vi "Get Team Ranking.vi"(11 "Needed Validations":u16) -> (3 "Ranked Teams":T1(array[cluster]))   [LabVIEW 2013]
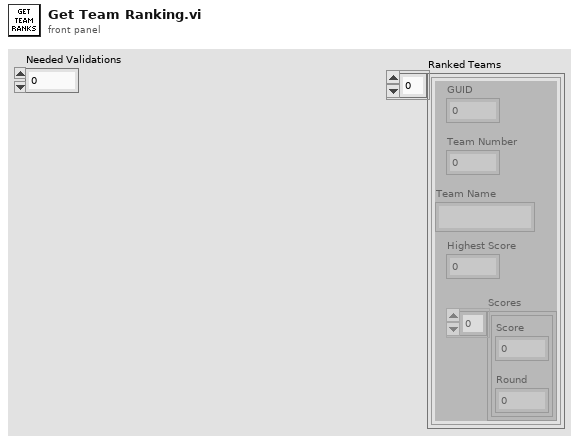
[diagram p1: front panel]
types:
  T1 = cluster{"GUID":u16, "Team Number":u16, "Team Name":string, "Highest Score":dbl, "Scores":cluster{"Score":dbl, "Round":u16}[]}[]
  T2 = cluster{"GUID":u16, "Team Number":u16, "Team Name":string, "Highest Score":dbl, "Scores":cluster{"Score":dbl, "Round":u16}[]}
  T3 = cluster{"Highest Score":dbl, "Scores":cluster{"Score":dbl, "Round":u16}[], "GUID":u16}[]
  T4 = typedef "ScoreList.ctl" = cluster{"ValidationCount":u16, "Score":T5}[]
  T5 = typedef "Full Score Entry.ctl" = cluster{"GUID":u16, "Score Mode Selector":u16, "Round Number":u16, "Full Score Entry":T6}
  T6 = typedef "ScoreEntry.ctl" = cluster{"Elements":cluster{"Name":string, "Value":string}[], "Score":dbl}
  T7 = cluster{"Highest Score":dbl, "Scores":cluster{"Score":dbl, "Round":u16}[], "GUID":u16}
  T8 = cluster{"Both":string, "Name":string, "GUID":u16, "Number":u16}
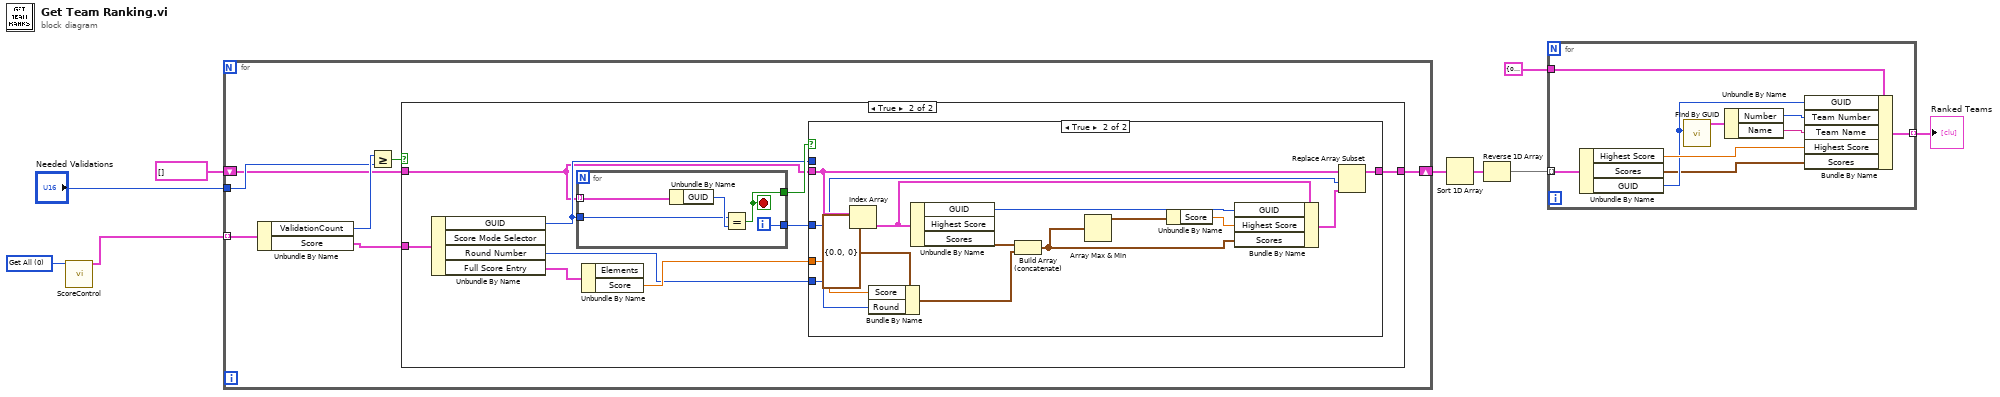
[diagram p0: block diagram]
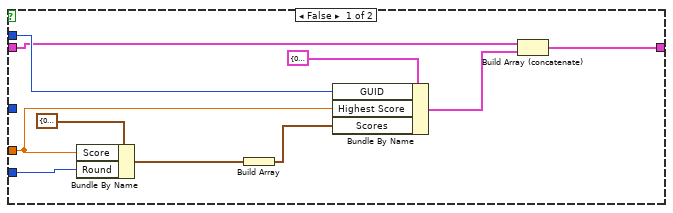
[diagram p3: hidden frame]
diagram:
  w2 = u16 0 items=["Get All", "Set", "Reset All", "Force Set"] ("Get/Set Mode Selector")
  n1 = call "ScoreControl.vi"("Get/Set Mode Selector"=w2) -> ("Scores"=w1:T4)  [unwired: 13 in, 1 out]
  n2 = for {
    tunnel: w1 -> [w16] mode=indexing
    tunnel: "Needed Validations" -> [w14]
    shift-right: [w10] -> w7
    shift-left: T3 [] -> [w11]
    n3 = Unbundle By Name(w16) -> ("ValidationCount"=w15:u16, "Score"=w12:T5)
    n4 = Greater Or Equal?(x=w15, y=w14) -> (x >= y?=w13:bool)
    n5 = case shown="True" w13 {
      tunnel: w12 -> [_ w26]
      tunnel: w11 -> [w17 w21]
      tunnel: [w17 w20] -> w10
      frame False {
      }
      frame True {
        n6 = Unbundle By Name(w26) -> ("GUID"=w24:u16, "Round Number"=w18:u16, "Full Score Entry"=w23:T6)  [unwired: 1 out]
        n7 = for {
          tunnel: w21 -> [w55] mode=indexing
          tunnel: w24 -> [w53]
          tunnel: [w52] -> w25
          tunnel: [w51] -> w19
          i -> [w51]
          stop <- w52 stop-if-true
          n8 = Unbundle By Name(w55) -> ("GUID"=w54:u16)
          n9 = Equal?(x=w53, y=w54) -> (x = y?=w52:bool)
        }
        n10 = Unbundle By Name(w23) -> ("Score"=w22:dbl)  [unwired: 1 out]
        n11 = case shown="True" w25 {
          tunnel: w24 -> [w35 _]
          tunnel: w22 -> [w29 w41]
          tunnel: w21 -> [w33 w47]
          tunnel: [w31 w44] -> w20
          tunnel: w19 -> [_ w46]
          tunnel: w18 -> [w28 w40]
          frame False {
            n12 = Bundle By Name(cluster=cluster{"Score":dbl, "Round":u16} {"Score"=0.0, "Round"=0}, "Score"=w29, "Round"=w28) -> (w27:cluster{"Score":dbl, "Round":u16})
            n13 = Build Array(w27) -> (w34:cluster{"Score":dbl, "Round":u16}[])
            n14 = Bundle By Name(cluster=T7 {"Highest Score"=0.0, "Scores"=[], "GUID"=0}, "GUID"=w35, "Highest Score"=w29, "Scores"=w34) -> (w32:T7)
            n15 = Build Array (concatenate)(w33, w32) -> (w31:T3)
          }
          frame True {
            n16 = Index Array(array=w47, index=w46) -> (element=w50:T7)
            n17 = Bundle By Name(cluster=cluster{"Score":dbl, "Round":u16} {"Score"=0.0, "Round"=0}, "Score"=w41, "Round"=w40) -> (w42:cluster{"Score":dbl, "Round":u16})
            n18 = Unbundle By Name(w50) -> ("GUID"=w49:u16, "Scores"=w37:cluster{"Score":dbl, "Round":u16}[])  [unwired: 1 out]
            n19 = Build Array (concatenate)(w37, w42) -> (w48:cluster{"Score":dbl, "Round":u16}[])
            n20 = Array Max & Min(array=w48) -> (max value=w39:cluster{"Score":dbl, "Round":u16})  [unwired: 3 out]
            n21 = Unbundle By Name(w39) -> ("Score"=w38:dbl)
            n22 = Bundle By Name(cluster=w50, "GUID"=w49, "Highest Score"=w38, "Scores"=w48) -> (w45:T7)
            n23 = Replace Array Subset(array=w47, new element=w45, index=w46) -> (w44:T3)
          }
        }
      }
    }
  }
  n24 = Sort 1D Array(array=w7) -> (sorted array=w4:T3)
  n25 = Reverse 1D Array(array=w4) -> (reversed array=w3:T3)
  n26 = for {
    tunnel: w3 -> [w64] mode=indexing
    tunnel: T2 {"GUID"=0, "Team Number"=0, "Team Name"="", "Highest Score"=0.0, "Scores"=[]} -> [w63]
    tunnel: [w57] -> w5 mode=indexing
    n27 = Unbundle By Name(w64) -> ("Highest Score"=w62:dbl, "Scores"=w56:cluster{"Score":dbl, "Round":u16}[], "GUID"=w61:u16)
    n28 = call "Find By GUID.vi"("GUID"=w61) -> ("Team"=w60:T8)  [unwired: 9 in, 1 out]
    n29 = Unbundle By Name(w60) -> ("Number"=w59:u16, "Name"=w58:string)
    n30 = Bundle By Name(cluster=w63, "GUID"=w61, "Team Number"=w59, "Team Name"=w58, "Highest Score"=w62, "Scores"=w56) -> (w57:T2)
  }
  "Ranked Teams" <- w5
